vi "Stop.vi"(8 "error in (no error)":errorcluster, 11 "IConfigure IAI in":refnum<class "IAI.lvclass">) -> (0 "error out":errorcluster, 3 "IConfigure IAI out":refnum<class "IAI.lvclass">)   [LabVIEW 2023, in "HAL Interfaces.lvlib" / "IAI.lvclass"]
uses:
  IAI.lvclass
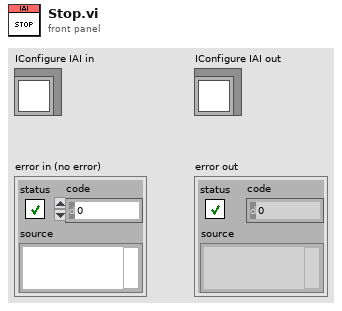
[diagram p1: front panel]
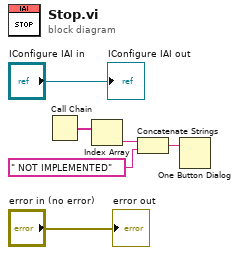
[diagram p0: block diagram]
diagram:
  n1 = Call Chain() -> (call chain=w4:string[])
  n2 = Index Array(array=w4) -> (element=w1:string)  [unwired: 1 in]
  n3 = Concatenate Strings(w1, " NOT IMPLEMENTED" ("string")) -> (w3:string)
  n4 = One Button Dialog(message=w3) -> ()  [unwired: 1 in, 1 out]
  "error out" <- "error in (no error)"
  "IConfigure IAI out" <- "IConfigure IAI in"
